vi "DualCam Field Position.vi"() -> (0 "Goal Found?":bool, 1 "Y":dbl, 3 "X":dbl, 4 "Gyro Angle":dbl)   [LabVIEW 2013]
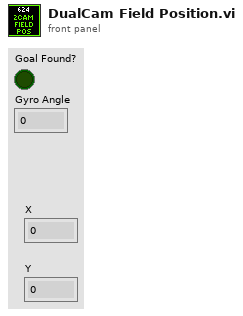
[diagram p1: front panel]
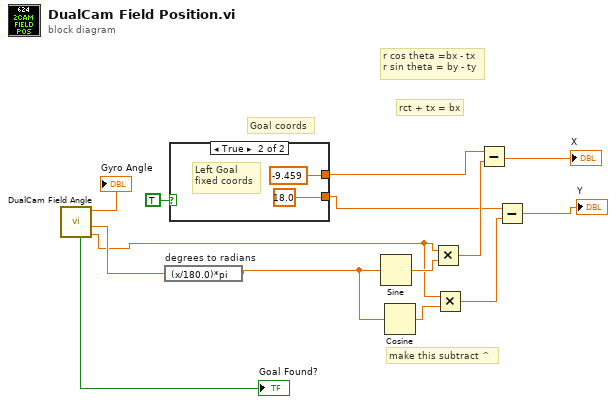
[diagram p0: block diagram]
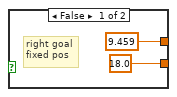
[diagram p2: hidden frame]
diagram:
  # "make this subtract ^"
  # "rct + tx = bx"
  # "r cos theta =bx - tx\nr sin theta = by - ty"
  # "Goal coords"
  n1 = call "DualCam Field Angle.vi"() -> ("LTarget Dist"=w4:dbl, "Field-Rel LTarget Angle"=w5:dbl, "Gyro Angle"=→"Gyro Angle":dbl, "Found?"=→"Goal Found?":bool)  [unwired: 8 in]
  n2 = expression code="(x/180.0)*pi" "degrees to radians"(w5) -> (w6:dbl)
  n3 = case shown="True" TRUE {
    tunnel: [9.459 -9.459] -> w12
    tunnel: [18.0 18.0] -> w7
    frame False {
      # "right goal\nfixed pos"
    }
    frame True {
      # "Left Goal\nfixed coords"
    }
  }
  n4 = Sine(x=w6) -> (sin(x)=w14:dbl)
  n5 = Cosine(x=w6) -> (cos(x)=w13:dbl)
  n6 = Multiply(x=w4, y=w14) -> (x*y=w11:dbl)
  n7 = Multiply(x=w4, y=w13) -> (x*y=w8:dbl)
  n8 = Subtract(x=w12, y=w11) -> (x-y=→"X":dbl)
  n9 = Subtract(x=w7, y=w8) -> (x-y=→"Y":dbl)
